vi "1011_FireEveryLastWednesdayInYearRange.vi"(8 "error in (no error)":errorcluster) -> (0 "error out":errorcluster)   [LabVIEW 2013]
uses:
  <vilib>/addons/_JKI Toolkits/Caraya/classes/Assert/Assert True.vi
  source/Cron/Create Cron Job.vi
  source/Cron/Compute Next Cron.vi
  source/Cron.Unix/Cron.Unix.lvclass
  <vilib>/addons/_JKI Toolkits/Caraya/classes/Test/Test.lvclass
  <vilib>/addons/_JKI Toolkits/Caraya/classes/Assert/Assert.lvclass
  source/openCron.lvlib
panel:
  out "Occurences":timestamp[](array[timestamp])
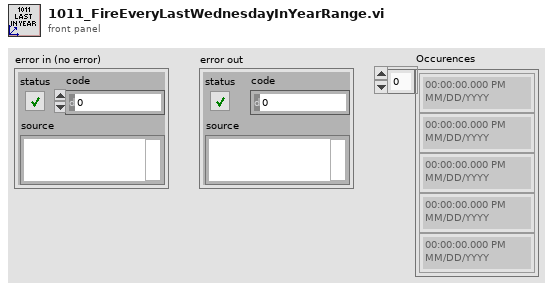
[diagram p1: front panel]
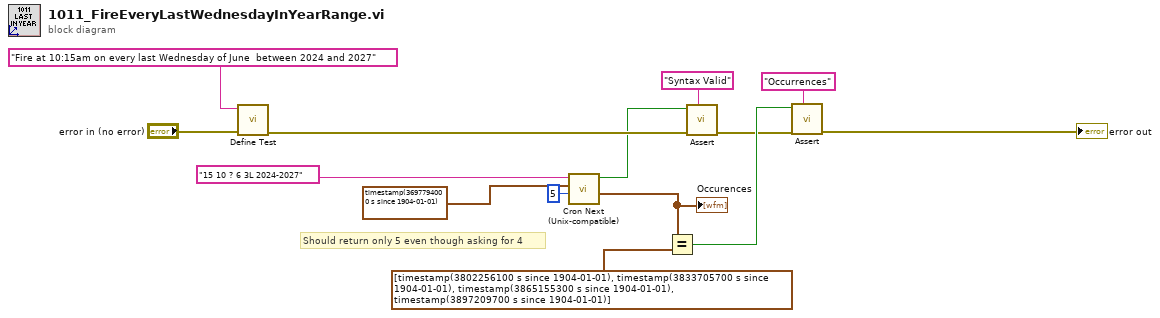
[diagram p0: block diagram]
diagram:
  # "Should return only 5 even though asking for 4"
  n1 = call <vilib>:"Define Test.vi"("error in (no error)"="error in (no error)", "Label (VI Title)"="Fire at 10:15am on every last Wednesday of June  between 2024 and 2027") -> ("error out"=w12:errorcluster)  [unwired: 9 in]
  n2 = call "Cron Next (Unix-compatible).vi"("Nb Occurences (min: 1)"=u16 5, "Reference timestamp (Now)"=timestamp(3697794000 s since 1904-01-01) ("y"), "Cron Expression"="15 10 ? 6 3L 2024-2027" ("Expression")) -> ("Occurences"=w8:timestamp[], "syntax valid?"=w9:bool)  [unwired: 6 in, 1 out]
  "Occurences" <- w8
  n3 = Equal?(x=w8, y=timestamp[] [timestamp(3802256100 s since 1904-01-01), timestamp(3833705700 s since 1904-01-01), timestamp(3865155300 s since 1904-01-01), timestamp(3897209700 s since 1904-01-01)]) -> (x = y?=w11:bool)
  n4 = call-poly <vilib>:"Assert.vi"("Label"="Syntax Valid" ("Label (VI Title)"), "error in (no error)"=w12, "True?"=w9) -> ("error out"=w10:errorcluster)  [unwired: 8 in]
  n5 = call-poly <vilib>:"Assert.vi"("Label"="Occurrences" ("Label (VI Title)"), "error in (no error)"=w10, "True?"=w11) -> ("error out"=→"error out":errorcluster)  [unwired: 8 in]
